vi "RFmx DPD Common Configuration.vi"(7 "Selector String":string, 8 "error in (no error)":errorcluster, 9 "Waveform":T1={"Waveform Name"="Wfm", "Waveform"={"x0"=0.0, "dx"=0.0, "y"=[]}, "Signal Bandwidth (Hz)"=0.0, "PAPR (dB)"=0.0, "Burst Length (s)"=0.0, "Sample Rate"=0.0, "Burst Start Locations"=[], "Burst Stop Locations"=[], "Idle Duration Present?"=FALSE, "Runtime Scaling"=0.0} {"Runtime Scaling" format="%#_6p"; "Sample Rate" format="%#_6p"; "Burst Length (s)" format="%#_6p"; "PAPR (dB)" format="%.2f"; "Signal Bandwidth (Hz)" format="%#_6p"; "Waveform"."y" format="%.2f"; "Waveform"."dx" format="%^.2e"; "Waveform"."x0" format="%^.2e"}, 10 "RFmx DPD Common Configuration":T2={"DPD Measurement Interval (s)"=0.0001, "Sample Rate Mode"=1, "Sample Rate (S/s)"=120000000.0, "Signal Type"=0, "Pre DPD CFR Enabled"=0, "Apply DPD CFR Enabled"=0, "DUT Average Input Power (dBm)"=-15.0} {"DUT Average Input Power (dBm)" format="%.2f"; "Apply DPD CFR Enabled" items=["False", "True"]; "Pre DPD CFR Enabled" items=["False", "True"]; "Signal Type" items=["Modulated", "Tones"]; "Sample Rate (S/s)" format="%.2p"; "Sample Rate Mode" items=["User", "Reference Waveform"]; "DPD Measurement Interval (s)" format="%#.2p"}, 11 "Instrument Handle In":refnum<k21>) -> (0 "error out":errorcluster, 3 "Instrument Handle Out":refnum<k21>)   [LabVIEW 2016, in "DPD.lvlib"]
uses:
  DPD.lvlib
  <vilib>/RFmx/SpecAn/mx/RFmxSpecAn.llb/RFmxSpecAn Select Measurement (Single).vi
  <resource>/objmgr/RFmxSpecAn.rc
  Typedefs/RFmx DPD Common Configuration.ctl
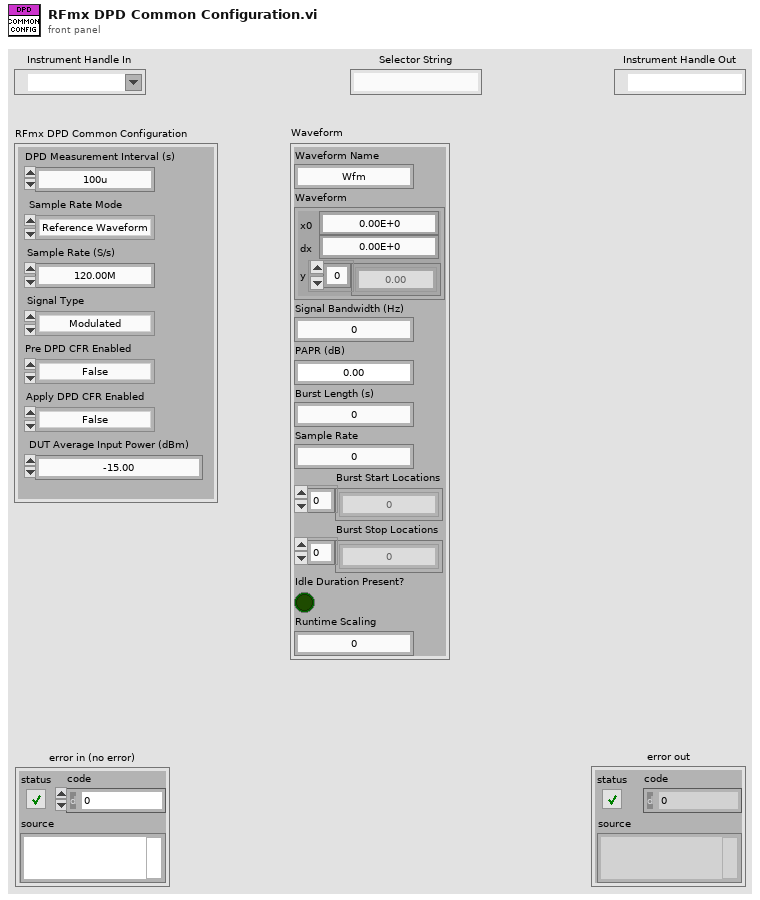
[diagram p1: front panel]
types:
  T1 = cluster{"Waveform Name":string, "Waveform":cluster{"x0":dbl, "dx":dbl, "y":csg[]}, "Signal Bandwidth (Hz)":dbl, "PAPR (dB)":dbl, "Burst Length (s)":dbl, "Sample Rate":dbl, "Burst Start Locations":i32[], "Burst Stop Locations":i32[], "Idle Duration Present?":bool, "Runtime Scaling":dbl}
  T2 = typedef "DPD.lvlib/RFmx DPD Common Configuration.ctl" = cluster{"DPD Measurement Interval (s)":dbl, "Sample Rate Mode":i32, "Sample Rate (S/s)":dbl, "Signal Type":i32, "Pre DPD CFR Enabled":i32, "Apply DPD CFR Enabled":i32, "DUT Average Input Power (dBm)":dbl}
  T3 = enum16{"ACP", "CCDF", "CHP", "FCnt", "Harmonics", "OBW", "SEM", "Spectrum", "Spur", "TXP", "AMPM", "DPD", "IQ", "IM", "NF", "PhaseNoise"}
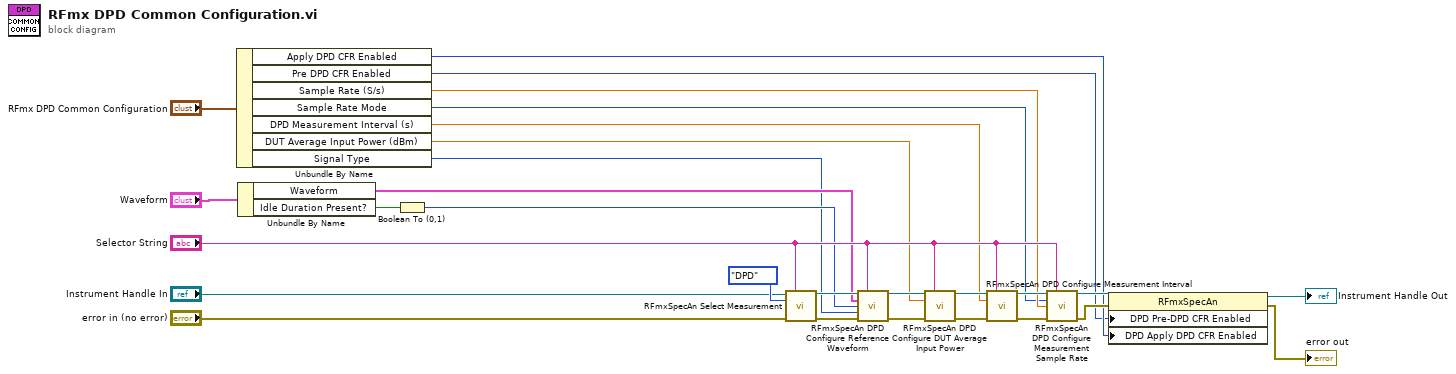
[diagram p0: block diagram]
diagram:
  n1 = Unbundle By Name("RFmx DPD Common Configuration") -> ("Apply DPD CFR Enabled"=w7:i32, "Pre DPD CFR Enabled"=w6:i32, "Sample Rate (S/s)"=w5:dbl, "Sample Rate Mode"=w4:i32, "DPD Measurement Interval (s)"=w3:dbl, "DUT Average Input Power (dBm)"=w2:dbl, "Signal Type"=w1:i32)
  n2 = Unbundle By Name("Waveform") -> ("Waveform"=w15:cluster{"x0":dbl, "dx":dbl, "y":csg[]}, "Idle Duration Present?"=w13:bool)
  n3 = Boolean To (0,1)(Boolean=w13) -> (0, 1=w12:i16)
  n4 = call-poly <vilib>:"RFmxSpecAn Select Measurement.vi"("Instrument Handle In"="Instrument Handle In", "Selector String"="Selector String", "Measurement"=T3."DPD", "error in (no error)"="error in (no error)") -> ("Instrument Handle Out"=w25:refnum<k21>, "error out"=w24:errorcluster)  [unwired: 10 in]
  n5 = call <vilib>:"RFmxSpecAn DPD Configure Reference Waveform.vi"("Instrument Handle In"=w25, "Selector String"="Selector String", "Reference Waveform"=w15, "Idle Duration Present"=w12, "Signal Type"=w1, "error in (no error)"=w24) -> ("Instrument Handle Out"=w23:refnum<k21>, "error out"=w22:errorcluster)  [unwired: 8 in]
  n6 = call <vilib>:"RFmxSpecAn DPD Configure DUT Average Input Power.vi"("Instrument Handle In"=w23, "Selector String"="Selector String", "DUT Average Input Power (dBm)"=w2, "error in (no error)"=w22) -> ("Instrument Handle Out"=w21:refnum<k21>, "error out"=w20:errorcluster)  [unwired: 10 in]
  n7 = call <vilib>:"RFmxSpecAn DPD Configure Measurement Interval.vi"("Instrument Handle In"=w21, "Selector String"="Selector String", "Measurement Interval (s)"=w3, "error in (no error)"=w20) -> ("Instrument Handle Out"=w19:refnum<k21>, "error out"=w18:errorcluster)  [unwired: 10 in]
  n8 = call <vilib>:"RFmxSpecAn DPD Configure Measurement Sample Rate.vi"("Instrument Handle In"=w19, "Selector String"="Selector String", "Sample Rate Mode"=w4, "Sample Rate (S/s)"=w5, "error in (no error)"=w18) -> ("Instrument Handle Out"=w9:refnum<k21>, "error out"=w8:errorcluster)  [unwired: 9 in]
  n9 = property class="RFmxSpecAn"(reference=w9, error in=w8, "DPD Pre-DPD CFR Enabled"=w6, "DPD Apply DPD CFR Enabled"=w7) -> (reference out=→"Instrument Handle Out":refnum<k21>, error out=→"error out":errorcluster)
